vi "PtbyPt Data Queue.vi"() -> ()   [LabVIEW 2013]
uses:
  <vilib>/ptbypt/NI_PtbyPt.lvlib
panel:
  in  "input data point":dbl format="%#_13g"
  in  "Boolean":bool
  in  "stop":bool
  out "Previous Queue":dbl[](array[numeric])
  out "Current Queue":dbl[](array[numeric])
  out "eliminated element":dbl format="%0.2f"
  out "current length":i32
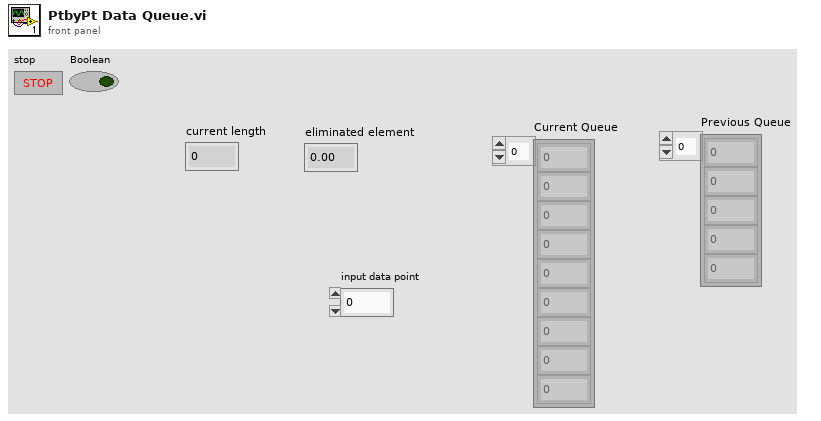
[diagram p1: front panel]
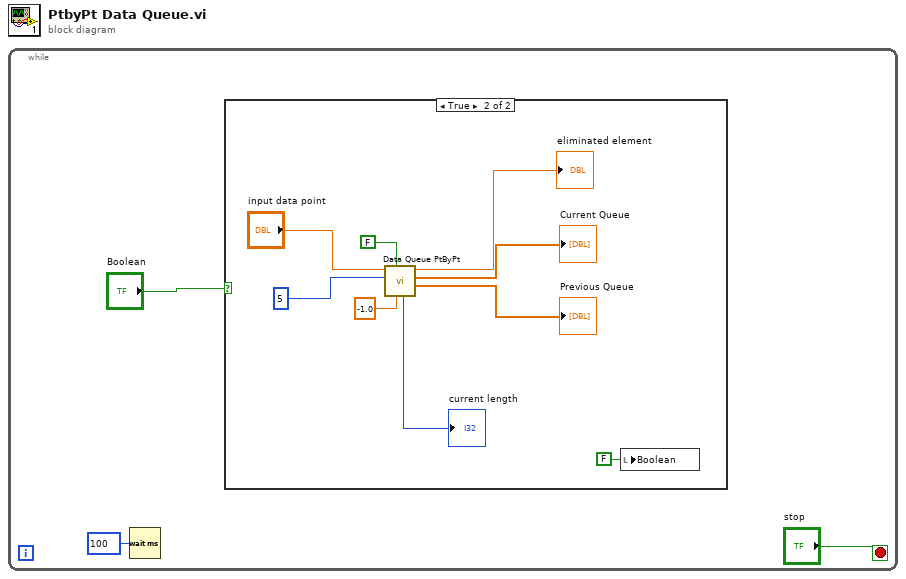
[diagram p0: block diagram]
diagram:
  n1 = while {
    stop <- "stop" stop-if-true
    n2 = Wait (ms)(milliseconds to wait=u32 100) -> ()  [unwired: 1 out]
    n3 = case shown="True" "Boolean" {
      frame False {
      }
      frame True {
        n4 = call <vilib>:"Data Queue PtByPt.vi"("initial queue element"=-1.0, "initialize"=FALSE, "sample length"=5, "input data point"="input data point") -> ("Previous Queue"=→"Previous Queue":dbl[], "Current Queue"=→"Current Queue":dbl[], "eliminated element"=→"eliminated element":dbl, "current length"=→"current length":i32)  [unwired: 3 in, 1 out]
        n5 = local write "Boolean"(FALSE ("Boolean")) -> ()
      }
    }
  }
